vi "OP400ZP_prep bdd conti.vi"(8 "tabin":string[](array[string]), 11 "contimaxin":string) -> (0 "tabout":string[](array[string]))   [LabVIEW 2020]
uses:
  OP400ZP_selectdata.ctl
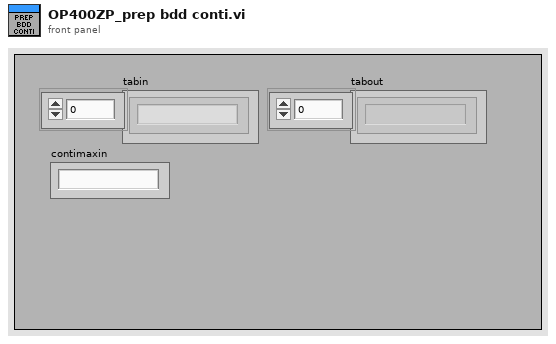
[diagram p1: front panel]
types:
  T1 = typedef "OP400ZP_selectdata.ctl" = u16
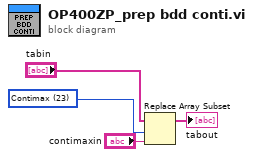
[diagram p0: block diagram]
diagram:
  w2 = T1 23 items=["IdOp400", "SN", "Type", "DateStart", "OCV", "ACIR", "InsuP", "InsuN", "TC0", "TC1", "DeltaTC", "VC0", "VC1", "DeltaVC", "MCU", "Tfactory", "RefLimite", "IniFileVers", "SoftVers", "ImageVers", "Pass", "Operateur", "TempsTest", "Contimax"] ("Menu déroulant")
  n1 = Replace Array Subset(array="tabin", new element="contimaxin", index=w2) -> (→"tabout":string[])
